vi "Read_VISA name.vi"(8 "error in (no error)":errorcluster, 11 "instrument in":refnum<class "instrument.lvclass">) -> (0 "error out":errorcluster, 2 "VISA resource name":refnum<visa-resource-name>, 3 "instrument out":refnum<class "instrument.lvclass">)   [LabVIEW 2018, in "instrument.lvclass"]
doc: "gets the \"VISA resource name\" of the object"
uses:
  instrument.lvclass
  instrument.lvclass/instrument.ctl
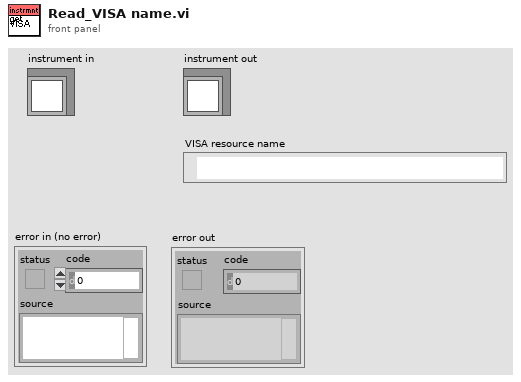
[diagram p1: front panel]
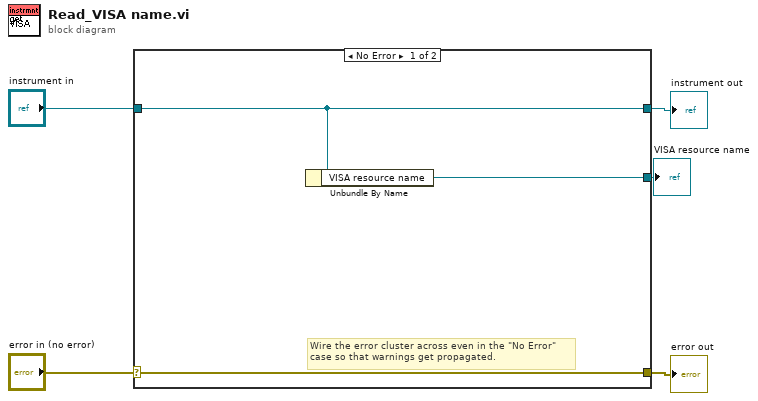
[diagram p0: block diagram]
diagram:
  n1 = case shown="No Error" "error in (no error)" {
    selector: "error in (no error)" -> [w8 w10]
    tunnel: [w8 w10] -> w4
    tunnel: [w7 w9] -> w2
    tunnel: "instrument in" -> [w7 w9]
    tunnel: [w6 _] -> w1
    frame No Error {
      # "Wire the error cluster across even in the \"No Error\"\ncase so that warnings get propagated."
      n2 = Unbundle By Name(w7) -> ("VISA resource name"=w6:refnum<visa-resource-name>)
    }
    frame Error {
    }
  }
  "error out" <- w4
  "instrument out" <- w2
  "VISA resource name" <- w1
